vi "Configure Dialog.vi"(2 "First time?":bool) -> ()   [LabVIEW 2016]
uses:
  Communication Global variables.vi
panel:
  in  "REST URL":string="http://192.168.3.204:5801"
  in  "Cancel Button":bool
  in  "Save":bool
  in  "UDP Port":u16=5803
  in  "Robot IP Address":string="10.27.67.2"
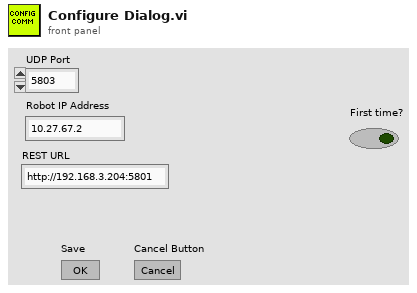
[diagram p1: front panel]
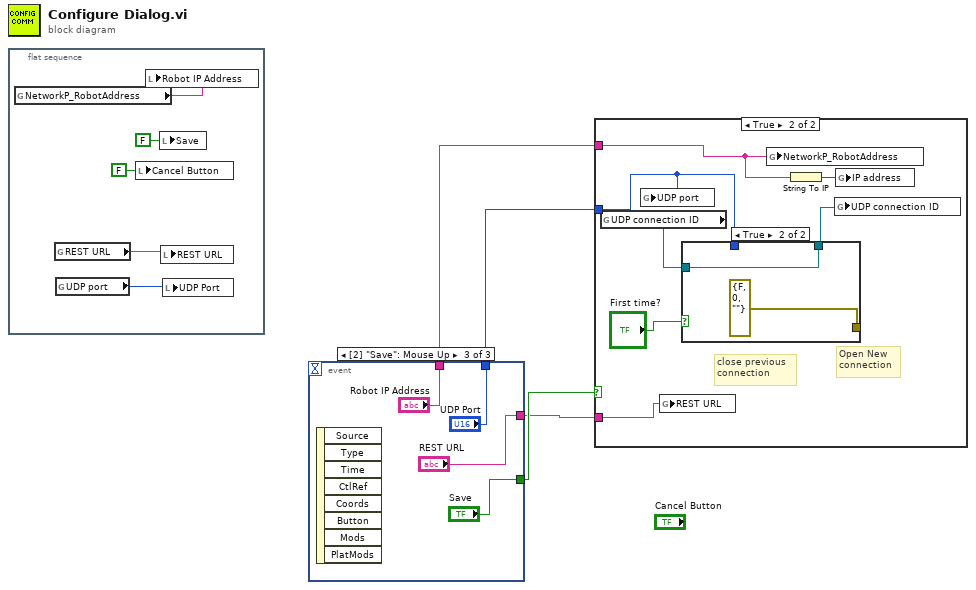
[diagram p0: block diagram]
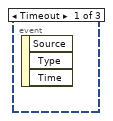
[diagram p2: hidden frame]
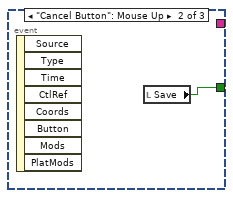
[diagram p3: hidden frame]
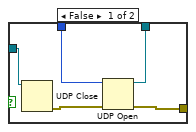
[diagram p5: hidden frame]
diagram:
  n1 = flat-sequence {
    frame #0 {
      n2 = global read "Communication Global variables.vi" "NetworkP_RobotAddress"() -> (w6:string)
      n3 = global read "Communication Global variables.vi" "REST URL"() -> (w5:string)
      n4 = global read "Communication Global variables.vi" "UDP port"() -> (w7:u16)
      n5 = local write "Cancel Button"(FALSE ("Cancel Button")) -> ()
      n6 = local write "Robot IP Address"(w6) -> ()
      n7 = local write "Save"(FALSE ("Save")) -> ()
      n8 = local write "REST URL"(w5) -> ()
      n9 = local write "UDP Port"(w7) -> ()
    }
  }
  n10 = event shown="[2] \"Save\": Mouse Up" {
    selector: _ -> [_ _ _]
    dyn-events: _ -> [_ _ _]
    timeout: _ -> [_ _ _]
    tunnel: [_ _ "Robot IP Address"] -> w4
    tunnel: [_ _ "UDP Port"] -> w3
    tunnel: [_ w10 "Save"] -> w2
    tunnel: [_ _ "REST URL"] -> w1
    event Timeout {
      n11 = event-data() -> ()  [unwired: 1 in, 3 out]
    }
    event "Cancel Button": Mouse Up {
      n12 = event-data() -> ()  [unwired: 1 in, 8 out]
      n13 = local read "Save"() -> (w10:bool)
    }
    event "Save": Mouse Up {
      n14 = event-data() -> ()  [unwired: 1 in, 8 out]
    }
  }
  n15 = case shown="True" w2 {
    tunnel: w3 -> [_ w16]
    tunnel: w4 -> [_ w15]
    tunnel: w1 -> [_ w19]
    frame False {
    }
    frame True {
      # "Open New \nconnection"
      # "close previous \nconnection"
      n16 = global read "Communication Global variables.vi" "UDP connection ID"() -> (w21:refnum<k16>)
      n17 = global write "Communication Global variables.vi" "UDP port"(w16) -> ()
      n18 = global write "Communication Global variables.vi" "REST URL"(w19) -> ()
      n19 = case shown="True" "First time?" {
        tunnel: w21 -> [w26 w27]
        tunnel: [w25 errorcluster {"status"=FALSE, "code"=0, "source"=""} ("error out")] -> _
        tunnel: [w23 w27] -> w17
        tunnel: w16 -> [w22 _]
        frame False {
          n20 = UDP Close(connection ID=w26) -> (error out=w24:errorcluster)  [unwired: 1 in, 1 out]
          n21 = UDP Open(8:w24, 11:w22) -> (port=w23:refnum<k16>, 0:w25:errorcluster)  [unwired: 3 in, 1 out]
        }
        frame True {
        }
      }
      n22 = global write "Communication Global variables.vi" "NetworkP_RobotAddress"(w15) -> ()
      n23 = String To IP(1:w15) -> (0:w20:u32)
      n24 = global write "Communication Global variables.vi" "UDP connection ID"(w17) -> ()
      n25 = global write "Communication Global variables.vi" "IP address"(w20) -> ()
    }
  }
